vi "Get Path Regex.vi"(8 "error in (no error)":errorcluster, 11 "Scores in":refnum<class "Scores.lvclass">) -> (0 "error out":errorcluster, 2 "Path Regex":string, 3 "Scores out":refnum<class "Scores.lvclass">)   [LabVIEW 2020, in "Scores.lvclass"]
uses:
  Scores.lvclass
  Scores.lvclass/Scores.ctl
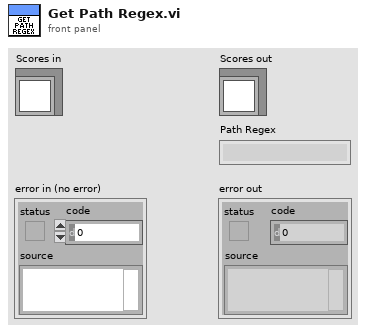
[diagram p1: front panel]
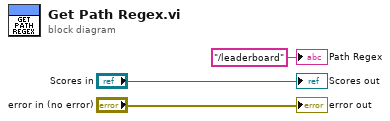
[diagram p0: block diagram]
diagram:
  "error out" <- "error in (no error)"
  "Scores out" <- "Scores in"
  "Path Regex" <- "/leaderboard" ("Path Regex")
